vi "Ex3Task3_SA.vi"() -> ()   [LabVIEW 2014]
panel:
  in  "stop":bool
  out "Moving Average":dbl
  out "Random Number":dbl
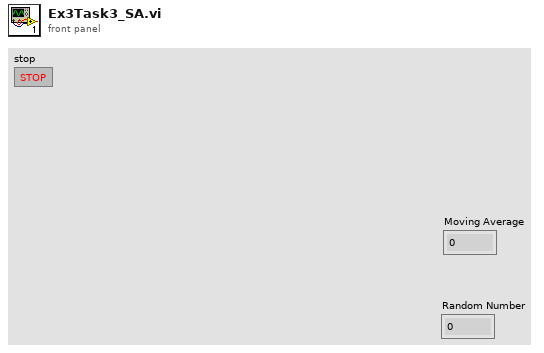
[diagram p1: front panel]
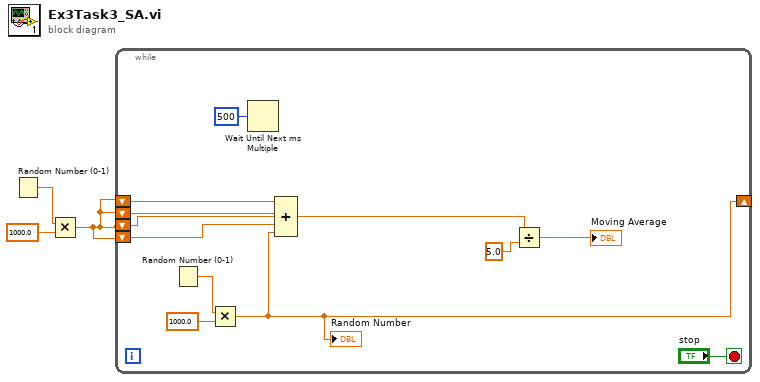
[diagram p0: block diagram]
diagram:
  n1 = Random Number (0-1)() -> (number: 0 to 1=w2:dbl)
  n2 = Multiply(x=w2, y=1000.0) -> (x*y=w1:dbl)
  n3 = while {
    shift-right: [w4] -> _
    shift-left: w1 -> [w10]
    shift-left: w1 -> [w7]
    shift-left: w1 -> [w8]
    shift-left: w1 -> [w9]
    stop <- "stop" stop-if-true
    n4 = Random Number (0-1)() -> (number: 0 to 1=w5:dbl)
    n5 = Multiply(x=w5, y=1000.0) -> (x*y=w4:dbl)
    "Random Number" <- w4
    n6 = Wait Until Next ms Multiple(millisecond multiple=u32 500) -> ()  [unwired: 1 out]
    n7 = Compound Arithmetic op=ADD(w10, w9, w8, w7, w4) -> (w12:dbl)
    n8 = Divide(x=w12, y=5.0) -> (x/y=→"Moving Average":dbl)
  }
